vi "classify error.vi"(8 "error to classify":errorcluster, 10 "attempt recovery?":bool, 11 "testmod runtime in":refnum<class "testmod runtime.lvclass">) -> (0 "classified error":errorcluster, 2 "error classification":T1, 3 "testmod runtime out":refnum<class "testmod runtime.lvclass">)   [LabVIEW 2013, in "testmod runtime.lvclass"]
doc: "Allows a module to classify an error generated at any point during execution. This <b>error classification</b> can then be used by calling code to determine if execution can continue. In addition, this function can be used to allow a component to clear an error, convert an error to a warning, or attempt to recover from an error. Recovery may be attempted only if <b>attempt recovery?</b> is true."
uses:
  testmod runtime.lvclass
  <vilib>/NI/Tag Bus Module Framework/runtime/error classification.ctl
  <vilib>/NI/Tag Bus Module Framework/runtime/TBM module execution interface.lvclass
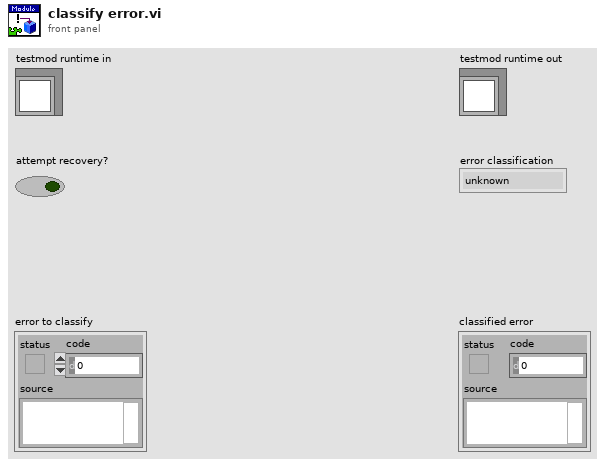
[diagram p1: front panel]
types:
  T1 = typedef "TBM module execution interface.lvclass/error classification.ctl" = enum16{"unknown", "none", "trivial", "recoverable", "critical"}
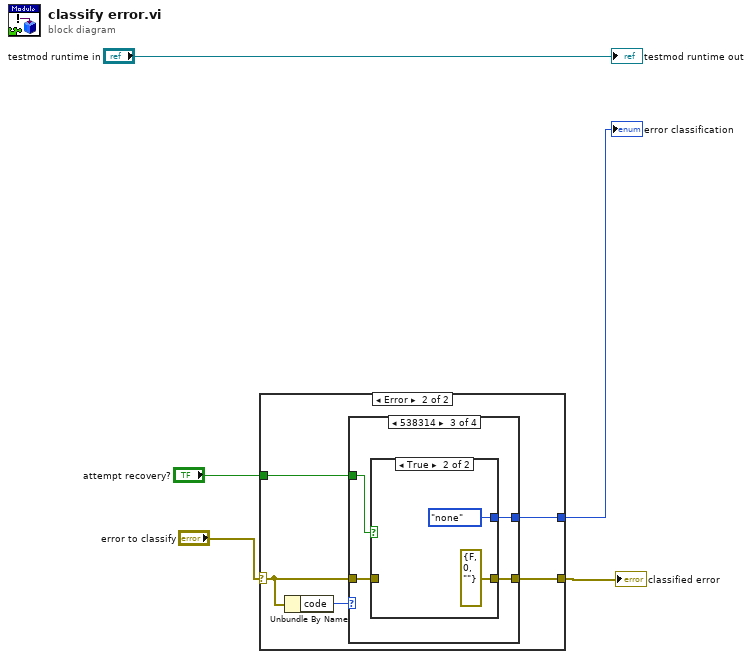
[diagram p0: block diagram]
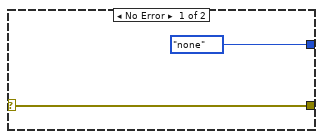
[diagram p2: hidden frame]
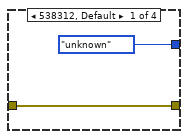
[diagram p3: hidden frame]
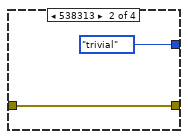
[diagram p4: hidden frame]
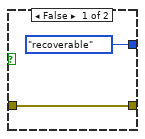
[diagram p5: hidden frame]
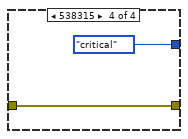
[diagram p6: hidden frame]
diagram:
  n1 = case shown="Error" "error to classify" {
    selector: "error to classify" -> [w7 w10]
    tunnel: [w7 w9] -> w4
    tunnel: [error_classification."none" ("error classification") w11] -> w2
    tunnel: "attempt recovery?" -> [_ w8]
    frame No Error {
    }
    frame Error {
      n2 = Unbundle By Name(w10) -> ("code"=w12:i32)
      n3 = case shown="538314" w12 {
        tunnel: [error_classification."unknown" ("error classification") error_classification."trivial" ("error classification") w20 error_classification."critical" ("error classification")] -> w11
        tunnel: w10 -> [w13 w15 w18 w25]
        tunnel: [w13 w15 w17 w25] -> w9
        tunnel: w8 -> [_ _ w19 _]
        frame 538312, Default {
        }
        frame 538313 {
        }
        frame 538314 {
          n4 = case shown="True" w19 {
            tunnel: [error_classification."recoverable" ("error classification") error_classification."none" ("error classification")] -> w20
            tunnel: w18 -> [w21 _]
            tunnel: [w21 errorcluster {"status"=FALSE, "code"=0, "source"=""} ("error IO")] -> w17
            frame False {
            }
            frame True {
            }
          }
        }
        frame 538315 {
        }
      }
    }
  }
  "error classification" <- w2
  "classified error" <- w4
  "testmod runtime out" <- "testmod runtime in"
